vi "AlazarAcqPrep.vi"(4 "TrigEnableMode":T5, 5 "Enable Trigger Enable":bool, 6 "rf lines per buffer":i32, 7 "Digitizer Settings":T1={"Digitizer delay (us) "=0.0, "rf points per line"=2048, "lines per plane"=128, "Samp Rate (Hz)"=100000000.0, "Additional dig delay (us)"=0.0, "Voltage Scale"=0.4, "Pre-Looks"=0, "Offset delay (us)"=0.0, "bits A/D"=8, "Avg Num"=1, "DigTimeOut"=5.0, "Rel Dig Delay"=0.0, "Dig Ch"=0, "LeCroyCluster"={"LeCroy Channels"=[TRUE, FALSE, FALSE, FALSE], "LC read pt offset"=0.0, "Sweep Avg"=FALSE}, "Main Digitizer"=enum."NI Digitizer", "Dig Config"=enum."Single channel", "Digitizer ID Cluster"={"Acqiris/Alazar/SP ID"=[], "NI Instr Handles"=[], "LeCroy VISA"="", "GaGe Handle"={"Handle"=0, "Sample size"=0, "Resolution"=0, "Offset"=0, "Channels"=0, "Boards"=0}, "ATS Ref"="ATS9350", "Acqiris Address"=["PCI::INSTR0"], "ADQRef"=refnum, "adq_cu_ptr"=refnum}, "Trigger Settings"={"Trig Source"=1, "Trig Coupling"=0, "Trig Slope"=0, "Level (mV)"=1500.0}, "Bulk Acq"=FALSE, "Bulk Start Indexes"=[], "Data Ref RF"=refnum, "NI ID/Channel"=[], "Total Dig CH"=1, "Xtra Ann Trig delay (us)"=10.0, "Fix Z Delay?"=FALSE, "One Way Transmission?"=FALSE, "Data Ref Log"=refnum} {"Trigger Settings"."Trig Slope" items=["Positive", "Negative"]; "Trigger Settings"."Level (mV)" format="%.2f"; "Trigger Settings"."Trig Coupling" items=["DC 1 MOhm", "AC 1 MOhm", "DC 50 Ohm", "AC 50 Ohm"]; "Trigger Settings"."Trig Source" items=["Chan 1", "External"]; "Rel Dig Delay" format="%.2f"; "DigTimeOut" format="%.2f"; "Avg Num" min=1; "Offset delay (us)" format="%.2f"; "Additional dig delay (us)" format="%.2f"; "Digitizer delay (us)" format="%.2f"}, 8 "BuffCount":i32=8, 9 "rf points per line":i32, 10 "AlazarDeviceIn":u32, 11 "Channel":i8) -> (1 "Return Code":u32, 2 "AlazarCluster":T6, 3 "DeviceOut":i32)   [LabVIEW 2022 SP3]
uses:
  C:/AlazarTech/ATS-VI/6.2.0/ATS_ctl/ATS_Async_Ctrl.ctl
  C:/AlazarTech/ATS-VI/6.2.0/ATS_ctl/ATS_Async_Mode.ctl
  C:/AlazarTech/ATS-VI/6.2.0/ATS_ctl/ATS_Async_Setting.ctl
  C:/AlazarTech/ATS-VI/6.2.0/ATS_ctl/ATS_Global_Ctrl.ctl
  C:/AlazarTech/ATS-VI/6.2.0/ATS_ctl/ATS_AuxOutSignal.ctl
  C:/AlazarTech/ATS-VI/6.2.0/ATS_ctl/ClockEdge.ctl
  C:/AlazarTech/ATS-VI/6.2.0/ATS_ctl/ATS_TriggerEnableMode.ctl
  -DigitizerRoutines/DigitizerSettings.ctl
  -DigitizerRoutines/DigitizerID.ctl
  -DigitizerRoutines/Digitizer.ctl
  -DigitizerRoutines/DigConfig.ctl
  C:/Windows/System32/ADQAPI_dotNet_helper.dll
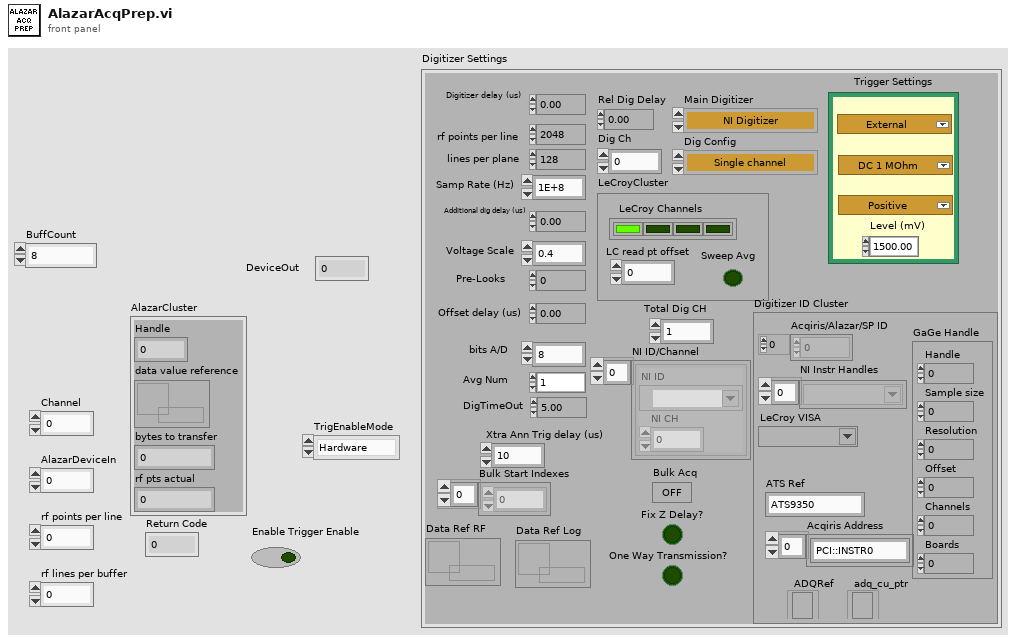
[diagram p1: front panel]
types:
  T1 = typedef "DigitizerSettings.ctl" = cluster{"Digitizer delay (us) ":dbl, "rf points per line":i32, "lines per plane":i32, "Samp Rate (Hz)":dbl, "Additional dig delay (us)":dbl, "Voltage Scale":dbl, "Pre-Looks":i32, "Offset delay (us)":dbl, "bits A/D":i8, "Avg Num":i32, "DigTimeOut":sgl, "Rel Dig Delay":sgl, "Dig Ch":i32, "LeCroyCluster":cluster{"LeCroy Channels":bool[], "LC read pt offset":dbl, "Sweep Avg":bool}, "Main Digitizer":T2, "Dig Config":T3, "Digitizer ID Cluster":T4, "Trigger Settings":cluster{"Trig Source":u16, "Trig Coupling":u16, "Trig Slope":u16, "Level (mV)":dbl}, "Bulk Acq":bool, "Bulk Start Indexes":i32[], "Data Ref RF":refnum<data-value>, "NI ID/Channel":cluster{"NI ID":refnum<k15>, "NI CH":i32}[], "Total Dig CH":i32, "Xtra Ann Trig delay (us)":dbl, "Fix Z Delay?":bool, "One Way Transmission?":bool, "Data Ref Log":refnum<data-value>}
  T2 = typedef "Digitizer.ctl" = enum16{"Acqiris Digitizer", "NI Digitizer", "LeCroy", "GaGe", "AlazarTech", "No Digitizer", "Teledyne"}
  T3 = typedef "DigConfig.ctl" = enum16{"Single channel", "2 Chans w/ 2 Acqiris", "2 Chans w/ 1 Acqiris", "5-CH Pulser New", "5-CH pulser w/ ann array", "5-pass style ann array", "Empty"}
  T4 = typedef "DigitizerID.ctl" = cluster{"Acqiris/Alazar/SP ID":u32[], "NI Instr Handles":refnum<k15>[], "LeCroy VISA":refnum<visa-resource-name>, "GaGe Handle":cluster{"Handle":u32, "Sample size":u32, "Resolution":i32, "Offset":i32, "Channels":u32, "Boards":u32}, "ATS Ref":string, "Acqiris Address":string[], "ADQRef":refnum<k24>, "adq_cu_ptr":refnum<k24>}
  T5 = typedef "ATS_TriggerEnableMode.ctl" = enum16{"Hardware", "Software"}
  T6 = cluster{"Handle":u32, "data value reference":refnum<data-value>, "bytes to transfer":u32, "rf pts actual":u32}
  T7 = typedef "ClockEdge.ctl" = u16
  T8 = typedef "ATS_Global_Ctrl.ctl" = enum16{"Init_Device", "Clear_ALL", "Set", "Get"}
  T9 = typedef "ATS_Async_Setting.ctl" = cluster{"UseHeader":u32, "Rec/Buffer":u32, "Total_Rec":u32, "DataBuffer":bool, "GetProcessedData":bool, "InterleaveSamples":bool}
  T10 = typedef "ATS_Async_Mode.ctl" = enum16{"Continuous", "Triggered", "No-Pre-Trigger", "Traditional"}
  T11 = typedef "ATS_Async_Ctrl.ctl" = enum16{"SetupDMA", "StartCapture", "Get", "Get_Stream", "Abort", "Stop"}
  T12 = typedef "Device_Info.ctl" = cluster{"Handle":u32, "Board":string, "CPLD":string, "MemorySize":u32, "SampleSize":u8, "ID":i32, "High_Memory":bool, "Chan/Board":u8}
  T13 = typedef "ATS_AuxOutSignal.ctl" = enum16{"Trigger Out", "Trigger Enable Out"}
  T14 = cluster{"Handle":u32, "data value reference":refnum<data-value>, u32, u32}
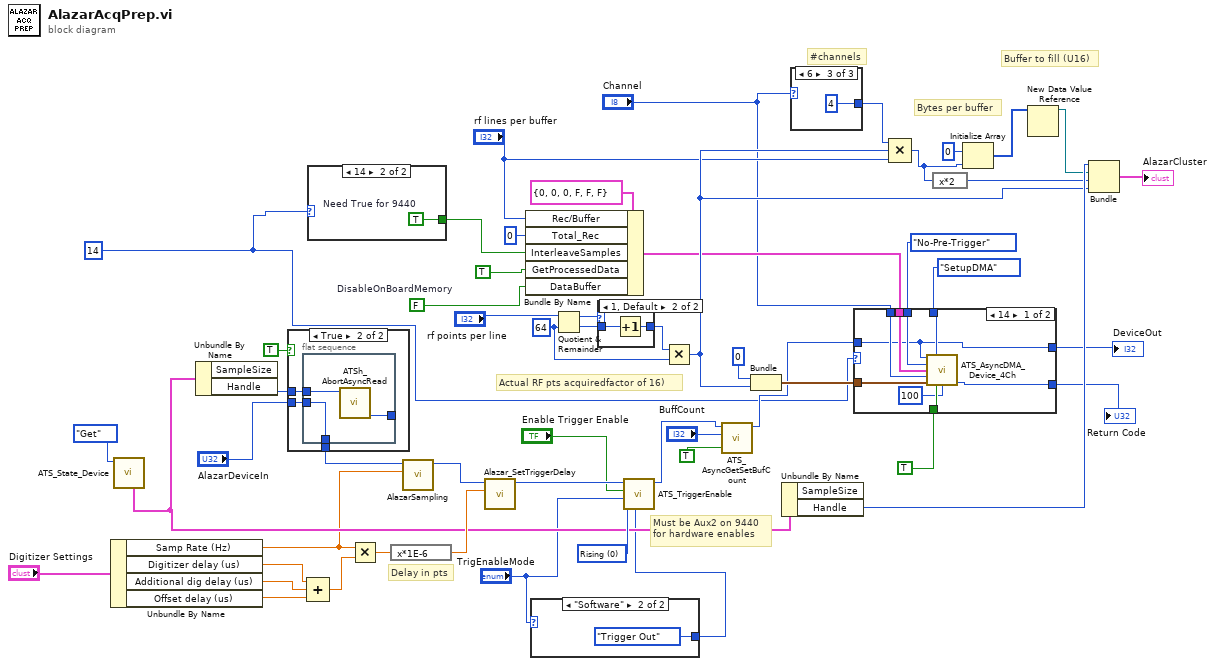
[diagram p0: block diagram]
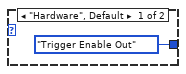
[diagram p5: hidden frame]
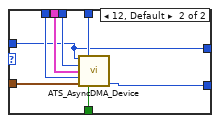
[diagram p6: hidden frame]
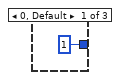
[diagram p7: hidden frame]
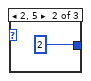
[diagram p8: hidden frame]
diagram:
  w1 = 14
  w27 = FALSE  # DisableOnBoardMemory
  w54 = T7 0 items=["Rising", "Falling"] ("AuxInSlope")
  w41 = u32 64 ("y")
  # "Must be Aux2 on 9440\nfor hardware enables"
  # "Actual RF pts acquiredfactor of 16)"
  # "Buffer to fill (U16)"
  # "Bytes per buffer"
  # "#channels"
  # "Delay in pts"
  n1 = Unbundle By Name("Digitizer Settings") -> ("Samp Rate (Hz)"=w11:dbl, "Digitizer delay (us)"=w15:dbl, "Additional dig delay (us)"=w14:dbl, "Offset delay (us)"=w13:dbl)
  n2 = call "ATS_State_Device.vi"("ATS_GBL_Ctrl"=ATS_Global_Ctrl."Get") -> ("DevInfo_Out"=w26:T12)  [unwired: 5 in, 5 out]
  n3 = Unbundle By Name(w26) -> ("Handle"=w25:u32)  [unwired: 1 out]
  n4 = case shown="True" TRUE {
    tunnel: [w55 w58] -> w28
    tunnel: w25 -> [_ w57]
    tunnel: "AlazarDeviceIn" -> [w55 w56]
    frame False {
    }
    frame True {
      n5 = flat-sequence {
        tunnel: w56 -> [w61]
        tunnel: [w61] -> w58
        tunnel: w57 -> [w60]
        tunnel: [w59] -> _
        frame #0 {
          n6 = call "ATSh_AbortAsyncRead.vi"("Handle"=w60) -> ("Return Code"=w59:u32)  [unwired: 10 in]
        }
      }
    }
  }
  n7 = Compound Arithmetic op=ADD(w15, w14, w13) -> (w10:dbl)
  n8 = case shown="14" w1 {
    tunnel: [_ w62] -> w8
    frame 0, Default {
    }
    frame 14 {
      w62 = TRUE  # Need True for 9440
    }
  }
  n9 = Multiply(x=w11, y=w10) -> (x*y=w39:dbl)
  n10 = expression code="x*1E-6"(w39) -> (w38:dbl)
  n11 = call "AlazarSampling.vi"("Sampling (Hz)"=w11, "DeviceIn"=w28) -> ("DeviceOut"=w53:i32)  [unwired: 8 in, 1 out]
  n12 = call "Alazar_SetTriggerDelay.vi"("Delay in Pts"=w38, "DeviceIn"=w53) -> ("DeviceOut"=w40:i32)  [unwired: 8 in, 1 out]
  n13 = Bundle By Name(cluster=T9 {"UseHeader"=0, "Rec/Buffer"=0, "Total_Rec"=0, "DataBuffer"=FALSE, "GetProcessedData"=FALSE, "InterleaveSamples"=FALSE} ("Async_Setting"), "Rec/Buffer"="rf lines per buffer", "Total_Rec"=u32 0, "InterleaveSamples"=w8, "GetProcessedData"=TRUE, "DataBuffer"=w27) -> (w36:T9)
  n14 = case shown="\"Software\"" "TrigEnableMode" {
    tunnel: [ATS_AuxOutSignal."Trigger Enable Out" ("AuxOutSignal") ATS_AuxOutSignal."Trigger Out" ("AuxOutSignal")] -> w23
    frame "Hardware", Default {
    }
    frame "Software" {
    }
  }
  n15 = Quotient & Remainder(x="rf points per line", y=w41) -> (x-y*floor(x/y)=w19:u32, floor(x/y)=w42:u32)
  n16 = case shown="1, Default" w19 {
    tunnel: [w65 w67] -> w44
    tunnel: w42 -> [w65 w66]
    frame 0 {
    }
    frame 1, Default {
      n17 = Increment(x=w66) -> (x+1=w67:u32)
    }
  }
  n18 = call "ATS_TriggerEnable.vi"("AuxOutSignal"=w23, "AuxInSlope"=w54, "TrigEnableMode"="TrigEnableMode", "Enable Trigger Enable"="Enable Trigger Enable", "Device"=w40) -> ("DeviceOut"=w5:i32)  [unwired: 5 in, 1 out]
  n19 = Multiply(x=w44, y=w41) -> (x*y=w49:u32)
  n20 = call "ATS_AsyncGetSetBufCount.vi"("Get / Set&Get"=TRUE, "BuffCount"="BuffCount", "DeviceIn"=w5) -> ("DeviceOut"=w4:i32)  [unwired: 6 in, 2 out]
  n21 = Bundle("Offset"=0, w49) -> (w34:cluster{"Offset":i32, u32})  [unwired: 1 in]
  n22 = Unbundle By Name(w26) -> ("Handle"=w51:u32)  [unwired: 1 out]
  n23 = case shown="6" "Channel" {
    tunnel: [u32 1 ("value") u32 2 ("value") u32 4 ("value")] -> w30
    frame 0, Default {
    }
    frame 2, 5 {
    }
    frame 6 {
    }
  }
  n24 = case shown="14" w1 {
    tunnel: w4 -> [w72 w80]
    tunnel: ATS_Async_Ctrl."SetupDMA" ("ATS_DMA_Ctrl") -> [w79 w87]
    tunnel: TRUE ("Start Now / Wait") -> [w74 w86]
    tunnel: w36 -> [w77 w85]
    tunnel: ATS_Async_Mode."No-Pre-Trigger" ("Async_Mode") -> [w78 w84]
    tunnel: w34 -> [w75 w83]
    tunnel: [w73 w82] -> w32
    tunnel: "Channel" -> [w76 w81]
    tunnel: [w72 w80] -> w3
    frame 14 {
      n25 = call "ATS_AsyncDMA_Device_4Ch.vi"("DeviceIn"=w72, "ATS_Async_Ctrl"=w79, "Async_Mode"=w78, "Async_Setting"=w77, "Channel"=w76, "ReadSamples"=w75, "Start Now / Wait"=w74, "WaitTimeOut (ms)"=u32 100) -> ("Return Code"=w73:u32)  [unwired: 3 in, 4 out]
    }
    frame 12, Default {
      n26 = call "ATS_AsyncDMA_Device.vi"("DeviceIn"=w80, "ATS_Async_Ctrl"=w87, "Async_Mode"=w84, "Async_Setting"=w85, "Channel"=w81, "ReadSamples"=w83, "Start Now / Wait"=w86) -> ("Return Code"=w82:u32)  [unwired: 4 in, 4 out]
    }
  }
  "Return Code" <- w32
  "DeviceOut" <- w3
  n27 = Compound Arithmetic op=MULTIPLY(w30, w49, "rf lines per buffer") -> (w47:u32)
  n28 = expression code="x*2"(w47) -> (w48:u32)
  n29 = Initialize Array(u16 0, w47) -> (w22:u16[])
  n30 = New Data Value Reference(data value=w22) -> (data value reference=w21:refnum<data-value>)  [unwired: 1 in, 1 out]
  n31 = Bundle("Handle"=w51, "data value reference"=w21, w48, w49) -> (→"AlazarCluster":T14)  [unwired: 1 in]
